vi "Loop_ACT_Drive.vi"() -> ()   [LabVIEW 2017]
uses:
  _SHARE ALL/RoboRio Share All/SRX Share All/TypeDefs SRX/Cluster_SRX_PIDF.ctl
  TypeDef/CLUSTER_Drive_HW_SRX_Status.ctl
  _SHARE ALL/RoboRio Share All/SRX Share All/TypeDefs SRX/Cluster_SRX_Common Runtime Data.ctl
  _SHARE ALL/RoboRio Share All/SRX Share All/TypeDefs SRX/Cluster_SRX_Error Calculations.ctl
  _SHARE ALL/RoboRio Share All/SRX Share All/TypeDefs SRX/Cluster_SRX_Voltage Out Data.ctl
  _SHARE ALL/RoboRio Share All/SRX Share All/TypeDefs SRX/Cluster_SRX_Sensor Out Data.ctl
  TypeDef/ENUM_Drive_ACT Loop_Mode.ctl
  TypeDef/CLUSTER_Left and Right.ctl
  cc483f24-0a62-4a22-b668-6104876bea72.vi
  Globals/Global_Device_IDs.vi
  _SHARE ALL/Global Share All/Global_STOP.vi
  Global_SM Write_Data Out.vi
  System Drivers/Phoenix-LabVIEW/Motor Controller/Get/CTRE_Phoenix_MotorController_GetAnalogData.vi
  Global_ACT Write_Data Out.vi
  WCDrive2018/WCDrive2018.lvlib
panel:
  in  "PIDF":T1={"P"=0.001, "I"=0.0, "D"=0.0, "F"=0.0, "I Zone"=1000.0}
  in  "Zero Encoder":bool
  out "Right Data":dbl
  out "Left Data":dbl
  out "Cycle Time (S)":dbl format="%.3g"
  in  "Target Time(ms)":u32=50
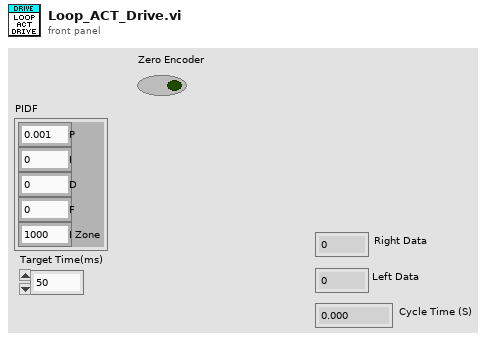
[diagram p1: front panel]
types:
  T1 = typedef "Cluster_SRX_PIDF.ctl" = cluster{"P":dbl, "I":dbl, "D":dbl, "F":dbl, "I Zone":dbl}
  T2 = typedef "CLUSTER_Left and Right.ctl" = cluster{"Left":dbl, "Right":dbl}
  T3 = typedef "ENUM_Drive_ACT Loop_Mode.ctl" = enum16{"Stop", "Position", "VBus", "Profile"}
  T4 = typedef "CLUSTER_Drive_HW_SRX_Status.ctl" = cluster{"Left":T5, "Right":T5}
  T5 = typedef "Cluster_SRX_Common Runtime Data.ctl" = cluster{"Calc":T6, "Voltage ":T7, "Sensor":T8, "Current":dbl, "Temp":dbl}
  T6 = typedef "Cluster_SRX_Error Calculations.ctl" = cluster{"Error":i32, "D-Error":dbl, "I-Acc":dbl}
  T7 = typedef "Cluster_SRX_Voltage Out Data.ctl" = cluster{"Percent":dbl, "Output":dbl, "Bus":dbl}
  T8 = typedef "Cluster_SRX_Sensor Out Data.ctl" = cluster{"Pos":i32, "Vel":i32}
  T9 = typedef "CLUSTER_Drive_Setup.ctl" = cluster{"Left Master":T10, "Right Master":T10, "Left Slave":T10, "Right Slave":T10, "Left Slave Top":T10, "Right Slave Top":T10}
  T10 = typedef "CLUSTER_Talon_Setup.ctl" = cluster{"Open Data":T11, "Current Config Data":T12, "Sensor Config":T13, "Hard Limits":T15, "Motion Magic Config Data":T17, "PIDF":T1, "Maximum Integral Accumulator Value":dbl, "AllowableClosedLoop":i32, "Limits":T18, "Output Config":T19}
  T11 = typedef "Cluster_SRX_OPEN Data.ctl" = cluster{"SRX ID":u8, "Invert Output":bool}
  T12 = typedef "Cluster_SRX_Current Config.ctl" = cluster{"Enable Current Limit?":bool, "Peak Current (Amps)":i32, "Peak Current Maximum Duration (ms)":i32, "Continuous Current Limit (Amps)":i32}
  T13 = typedef "Cluster_SRX_Sensor Config.ctl" = cluster{"Feedback Device":T14, "PhaseSensor":bool}
  T14 = typedef "CTRE_Phoenix_MotorControl_FeedbackDevice.ctl" = i8
  T15 = typedef "Cluster_SRX_Config Hard Limits.ctl" = cluster{"Fwd Enable":bool, "Rev Enable":bool, "Fwd NO-NC":T16, "Rev NO-NC":T16}
  T16 = typedef "CTRE_Phoenix_MotorControl_LimitSwitchNormal.ctl" = enum16{"Normally Open", "Normally Closed", "Disabled"}
  T17 = typedef "Cluster_SRX_Motion Magic Config Data.ctl" = cluster{"Cruise Velocity":i32, "Acceleration":i32}
  T18 = typedef "Cluster_SRX_Config Soft Limits.ctl" = cluster{"Max":i32, "Min":i32, "Max Enable":bool, "Min Enable":bool}
  T19 = typedef "Cluster_SRX_Config Voltage Output.ctl" = cluster{"Invert?":bool, "Neutral Mode":T20, "Deadband (-1to1)":dbl, "Ramp Time Off to Full (S)":dbl, "Peak  (-1to1)":T21, "Nominal  (-1to1)":T21}
  T20 = typedef "CTRE_Phoenix_MotorControl_NeutralMode.ctl" = enum8{"EEPROMSetting", "Override to Coast", "Override to Brake"}
  T21 = typedef "Cluster_SRX_Forward and Reverse.ctl" = cluster{"Forward":dbl, "Reverse":dbl}
  T22 = typedef "WPI_RobotDriveDevRef.ctl" = cluster{"DevStatus":errorcluster, "Motors[]":T23[], "Square Inputs":bool, "Max Output":dbl}
  T23 = typedef "WPI_MotorControlDeviceRef.ctl" = cluster{"DeviceStatus":errorcluster, "Type":T24, "PWM":cluster{"PWM Channel":T25, "DeadBand":T26}, "CAN":cluster{"Device Number":u8, "SetOutput VI Ref":variant, "GetOutput VI Ref":variant, "Enable VI Ref":variant, "Disable VI Ref":variant, "Data":variant}, "Invert":bool, "DIO PWM":cluster{"PWM \"Enable\" Channel":T25, "DIOChannel":T27, "PWM Rate":dbl}}
  T24 = typedef "WPI_MotorControlType.ctl" = enum16{"PWM", "CAN", "DIO PWM"}
  T25 = typedef "FPGA_DIOPWMChannel.ctl" = enum8{"PWM 0", "PWM 1", "PWM 2", "PWM 3", "PWM 4", "PWM 5", "PWM 6", "PWM 7", "PWM 8", "PWM 9", "PWM MXP 0", "PWM MXP 1", "PWM MXP 2", "PWM MXP 3", "PWM MXP 4", "PWM MXP 5", "PWM MXP 6", "PWM MXP 7", "PWM MXP 8", "PWM MXP 9", "Invalid"}
  T26 = typedef "WPI_PWMDeadband.ctl" = cluster{"Name":string, "maxPositivePwm":i32, "minPositivePwm":i32, "centerPwm":i32, "maxNegativePwm":i32, "minNegativePwm":i32, "angularRange":u16}
  T27 = typedef "FPGA_DIOChannel.ctl" = enum8{"DIO 0", "DIO 1", "DIO 2", "DIO 3", "DIO 4", "DIO 5", "DIO 6", "DIO 7", "DIO 8", "DIO 9", "DIO MXP 0", "DIO MXP 1", "DIO MXP 2", "DIO MXP 3", "DIO MXP 4", "DIO MXP 5", "DIO MXP 6", "DIO MXP 7", "DIO MXP 8", "DIO MXP 9", "DIO MXP 10", "DIO MXP 11", "DIO MXP 12", "DIO MXP 13", "DIO MXP 14", "DIO MXP 15", "SPI Port CS1", "SPI Port CS2", "SPI Port CS3", "SPI Port MISO", "SPI Port MOSI", "Invalid"}
  T28 = cluster{"RobotDriveDevRef Out":T22, "Target Time(ms)":u32, "Current Time":timestamp, "Previous Time":timestamp, "Cycle Time (S)":dbl, "SRX_Status":T4, "Mode":T3, "VBus":T2, "Cruise RPM":dbl, "MAX Velocity\n":dbl, "Encoder Target Position":i32, "Zero Encoder":bool}
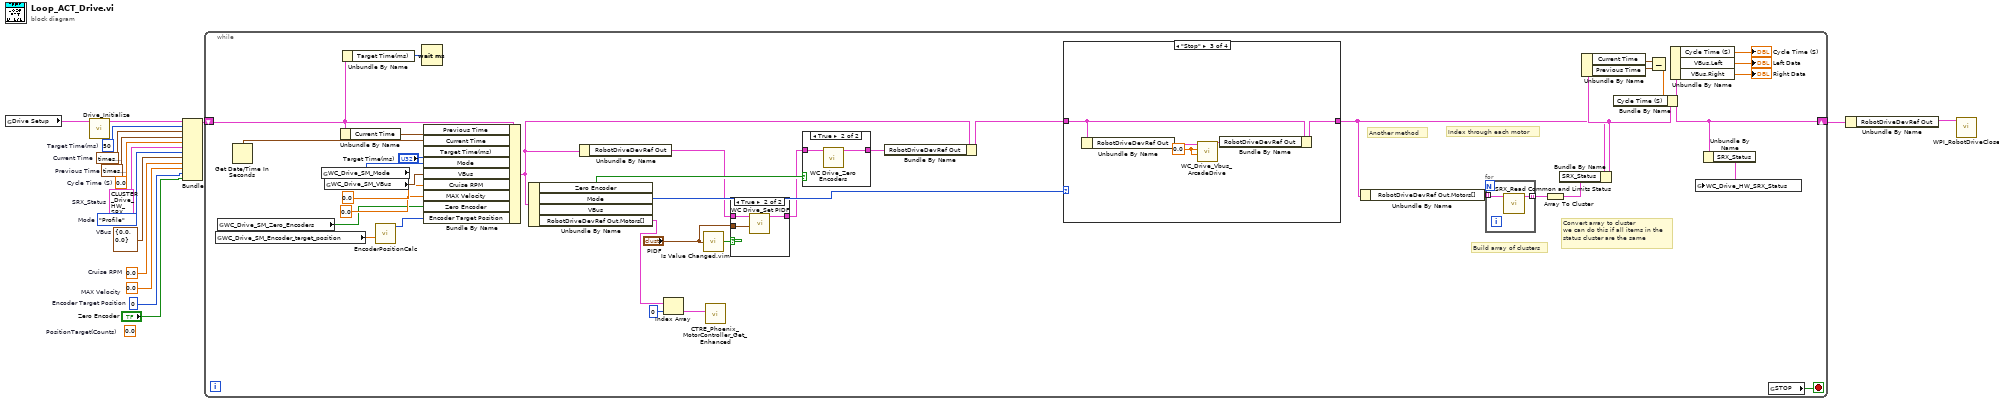
[diagram p0: block diagram]
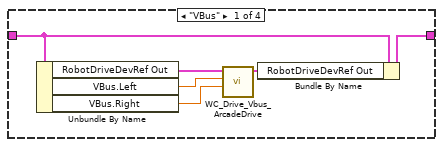
[diagram p4: hidden frame]
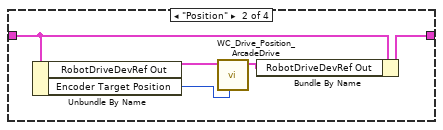
[diagram p5: hidden frame]
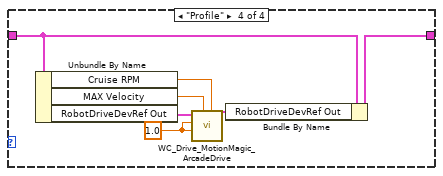
[diagram p6: hidden frame]
diagram:
  (unwired) 0.0  # PositionTarget(Counts)
  w4 = 0  # Encoder Target Position
  w5 = 0.0  # MAX Velocity
  w6 = 0.0  # Cruise RPM
  w7 = T2 {"Left"=0.0, "Right"=0.0}  # VBus
  w8 = ENUM_Drive_ACT_Loop_Mode."Profile"  # Mode
  w9 = T4 {"Left"={"Calc"={"Error"=0, "D-Error"=0.0, "I-Acc"=0.0}, "Voltage "={"Percent"=0.0, "Output"=0.0, "Bus"=0.0}, "Sensor"={"Pos"=0, "Vel"=0}, "Current"=0.0, "Temp"=0.0}, "Right"={"Calc"={"Error"=0, "D-Error"=0.0, "I-Acc"=0.0}, "Voltage "={"Percent"=0.0, "Output"=0.0, "Bus"=0.0}, "Sensor"={"Pos"=0, "Vel"=0}, "Current"=0.0, "Temp"=0.0}}  # SRX_Status
  w11 = 0.0  # Cycle Time (S)
  w16 = timestamp(0 s since 1904-01-01)  # Previous Time
  w15 = timestamp(0 s since 1904-01-01)  # Current Time
  w14 = u32 50  # Target Time(ms)
  n1 = global read "Global_Device_IDs.vi" "Drive Setup"() -> (w1:T9)
  n2 = call "Drive_Initialize.vi"("Drive Setup"=w1) -> ("RobotDriveDevRef Out"=w3:T22)  [unwired: 10 in]
  n3 = Bundle("RobotDriveDevRef Out"=w3, "Target Time(ms)"=w14, "Current Time"=w15, "Previous Time"=w16, "Cycle Time (S)"=w11, "SRX_Status"=w9, "Mode"=w8, "VBus"=w7, "Cruise RPM"=w6, "MAX Velocity"=w5, "Encoder Target Position"=w4, "Zero Encoder"="Zero Encoder") -> (w13:T28)  [unwired: 1 in]
  n4 = while {
    shift-right: [w40] -> w12
    shift-left: w13 -> [w37]
    stop <- w54 stop-if-true
    # "Build array of clusters"
    # "Convert array to cluster\nwe can do this if all items in the\nstatus cluster are the same"
    # "Index through each motor"
    # "Another method"
    n5 = global read "Global_SM Write_Data Out.vi" "WC_Drive_SM_Encoder_target_position"() -> (w31:dbl)
    n6 = global read "Global_SM Write_Data Out.vi" "WC_Drive_SM_Zero_Encoders"() -> (w33:bool)
    n7 = Get Date/Time In Seconds() -> (seconds since 1Jan1904=w53:timestamp)
    n8 = global read "Global_SM Write_Data Out.vi" "WC_Drive_SM_Mode"() -> (w43:T3)
    n9 = global read "Global_SM Write_Data Out.vi" "WC_Drive_SM_VBus"() -> (w36:T2)
    n10 = Unbundle By Name(w37) -> ("Current Time"=w52:timestamp)
    n11 = Unbundle By Name(w37) -> ("Target Time(ms)"=w48:u32)
    n12 = call "EncoderPositionCalc.vi"("PositionTarget(in)"=w31) -> ("PostionTarget(Counts)"=w32:i32)  [unwired: 10 in]
    n13 = Wait (ms)(milliseconds to wait=w48) -> ()  [unwired: 1 out]
    n14 = Bundle By Name(cluster=w37, "Previous Time"=w52, "Current Time"=w53, "Target Time(ms)"="Target Time(ms)", "Mode"=w43, "VBus"=w36, "Cruise RPM"=0.0, "MAX Velocity"=0.0, "Zero Encoder"=w33, "Encoder Target Position"=w32) -> (w22:T28)
    n15 = Unbundle By Name(w22) -> ("Zero Encoder"=w27:bool, "Mode"=w42:T3, "RobotDriveDevRef Out.Motors[]"=w19:T23[])  [unwired: 1 out]
    n16 = Unbundle By Name(w22) -> ("RobotDriveDevRef Out"=w24:T22)
    n17 = Index Array(array=w19, index=0) -> (element=w17:T23)
    n18 = call "Is Value Changed.vim"("value"="PIDF") -> ("changed or first call?"=w25:bool)
    n19 = call-poly "CTRE_Phoenix_MotorController_Get_Enhanced.vi"("PhoenixMotorControlDevRef"=w17) -> ()  [unwired: 10 in, 5 out]
    n20 = case shown="True" w25 {
      tunnel: "PIDF" -> [_ w58]
      tunnel: w24 -> [w55 w57]
      tunnel: [w55 w56] -> w23
      frame False {
      }
      frame True {
        n21 = call "WC Drive_Set PIDF.vi"("PIDF"=w58, "RobotDriveDevRef"=w57) -> ("RobotDriveDevRef Out"=w56:T22)  [unwired: 8 in, 1 out]
      }
    }
    n22 = case shown="True" w27 {
      tunnel: w23 -> [w59 w61]
      tunnel: [w59 w60] -> w20
      frame False {
      }
      frame True {
        n23 = call "WC Drive_Zero Encoders.vi"("RobotDriveDevRef"=w61) -> ("RobotDriveDevRef Out"=w60:T22)  [unwired: 9 in, 1 out]
      }
    }
    n24 = Bundle By Name(cluster=w22, "RobotDriveDevRef Out"=w20) -> (w21:T28)
    n25 = case shown="\"Stop\"" w42 {
      tunnel: w21 -> [w65 w74 w78 w82]
      tunnel: [w64 w73 w77 w83] -> w38
      frame "VBus" {
        n26 = Unbundle By Name(w65) -> ("RobotDriveDevRef Out"=w69:T22, "VBus.Left"=w68:dbl, "VBus.Right"=w67:dbl)
        n27 = call "WC_Drive_Vbus_ArcadeDrive.vi"("Right Value"=w67, "Left Value"=w68, "RobotDriveDevRef"=w69) -> ("RobotDriveDevRef Out"=w66:T22)  [unwired: 7 in, 1 out]
        n28 = Bundle By Name(cluster=w65, "RobotDriveDevRef Out"=w66) -> (w64:T28)
      }
      frame "Position" {
        n29 = Unbundle By Name(w74) -> ("RobotDriveDevRef Out"=w72:T22, "Encoder Target Position"=w70:i32)
        n30 = call "WC_Drive_Position_ArcadeDrive.vi"("Encoder Target Position"=w70, "RobotDriveDevRef"=w72) -> ("RobotDriveDevRef Out"=w71:T22)  [unwired: 8 in, 1 out]
        n31 = Bundle By Name(cluster=w74, "RobotDriveDevRef Out"=w71) -> (w73:T28)
      }
      frame "Stop" {
        w76 = 0.0 ("X axis value")
        n32 = Unbundle By Name(w78) -> ("RobotDriveDevRef Out"=w75:T22)
        n33 = call "WC_Drive_Vbus_ArcadeDrive.vi"("Right Value"=w76, "Left Value"=w76, "RobotDriveDevRef"=w75) -> ("RobotDriveDevRef Out"=w79:T22)  [unwired: 7 in, 1 out]
        n34 = Bundle By Name(cluster=w78, "RobotDriveDevRef Out"=w79) -> (w77:T28)
      }
      frame "Profile" {
        w85 = 1.0 ("X axis value")
        n35 = Unbundle By Name(w82) -> ("Cruise RPM"=w81:dbl, "MAX Velocity"=w80:dbl, "RobotDriveDevRef Out"=w86:T22)
        n36 = call "WC_Drive_MotionMagic_ArcadeDrive.vi"("Cruise RPM"=w81, "Max Velocity"=w80, "Right Value"=w85, "Left Value"=w85, "RobotDriveDevRef"=w86) -> ("RobotDriveDevRef Out"=w84:T22)  [unwired: 5 in, 1 out]
        n37 = Bundle By Name(cluster=w82, "RobotDriveDevRef Out"=w84) -> (w83:T28)
      }
    }
    n38 = Unbundle By Name(w38) -> ("RobotDriveDevRef Out.Motors[]"=w30:T23[])
    n39 = for {
      tunnel: w30 -> [w63] mode=indexing
      tunnel: [w62] -> w29 mode=indexing
      n40 = call "SRX_Read Common and Limits Status.vi"("PhoenixMotorControlDevRef"=w63) -> ("Common Runtime Data Out"=w62:T5)  [unwired: 8 in, 2 out]
    }
    n41 = Array To Cluster(array=w29) -> (cluster=w28:cluster{"[0]":T5, "[1]":T5})
    n42 = Bundle By Name(cluster=w38, "SRX_Status"=w28) -> (w39:T28)
    n43 = Unbundle By Name(w39) -> ("Current Time"=w51:timestamp, "Previous Time"=w50:timestamp)
    n44 = Subtract(x=w51, y=w50) -> (x-y=w41:dbl)
    n45 = Bundle By Name(cluster=w39, "Cycle Time (S)"=w41) -> (w40:T28)
    n46 = Unbundle By Name(w40) -> ("Cycle Time (S)"=→"Cycle Time (S)":dbl, "VBus.Left"=→"Left Data":dbl, "VBus.Right"=→"Right Data":dbl)
    n47 = Unbundle By Name(w40) -> ("SRX_Status"=w44:T4)
    n48 = global write "Global_ACT Write_Data Out.vi" "WC_Drive_HW_SRX_Status"(w44) -> ()
    n49 = global read "Global_STOP.vi" "STOP"() -> (w54:bool)
  }
  n50 = Unbundle By Name(w12) -> ("RobotDriveDevRef Out"=w10:T22)
  n51 = call <vilib>:"WPI_RobotDriveClose.vi"("RobotDriveDevRef"=w10) -> ()  [unwired: 10 in, 1 out]
